vi "N4_201_Adjust.vi"(4 "Driver Name":T10, 5 "ValueIn":T7, 6 "Error Code":T11, 7 "Command":T7, 8 "error in":T9, 11 "DriverConnect in":T1={"InterfaceType"=enum."VISA", "OpenedSession"="", "InterfaceSettings"={"Interface"=enum."RS232", "EOS 4 read"=enum."LF (\\n)", "EOS 4 write"=enum."LF (\\n)", "TMO, ms"=10000, "Sett"=variant(cluster{"Baud Rate":u32, "Data Bits":u16, "Parity":u16, "Stop Bits":u16, "Flow Control":u16, "Eho":bool} {"Baud Rate"=75, "Data Bits"=0, "Parity"=0, "Stop Bits"=0, "Flow Control"=0, "Eho"=FALSE})}}) -> (0 "error out":T9, 3 "DriverConnect out":T1={"InterfaceType"=enum."VISA", "OpenedSession"="", "InterfaceSettings"={"Interface"=enum."RS232", "EOS 4 read"=enum."LF (\\n)", "EOS 4 write"=enum."LF (\\n)", "TMO, ms"=10000, "Sett"=variant(cluster{"Baud Rate":u32, "Data Bits":u16, "Parity":u16, "Stop Bits":u16, "Flow Control":u16, "Eho":bool} {"Baud Rate"=75, "Data Bits"=0, "Parity"=0, "Stop Bits"=0, "Flow Control"=0, "Eho"=FALSE})}})   [LabVIEW 2018]
uses:
  MOKO_LabViewLibrary/MokoLowLevel/MokoLowLovelControl/MLLC_ErrorCode.ctl
  MOKO_LabViewLibrary/MokoLowLevel/MokoLowLovelControl/MLLC_DriverName.ctl
  MOKO_LabViewLibrary/MokoLowLevel/MokoLowLovelControl/MLLC_Error.ctl
  MOKO_LabViewLibrary/MokoLowLevel/MokoLowLovelControl/MLLC_Boolean.ctl
  MOKO_LabViewLibrary/MokoLowLevel/MokoLowLovelControl/MLLC_Command.ctl
  MOKO_LabViewLibrary/MokoLowLevel/MokoLowLovelControl/MLLC_Delay.ctl
  MOKO_LabViewLibrary/MokoLowLevel/MokoLowLovelControl/MLLC_ConnectCluster.ctl
  MOKO_LabViewLibrary/MokoLowLevel/MokoLowLovelControl/MLLC_InterfaceType.ctl
  MOKO_LabViewLibrary/MokoLowLevel/MokoLowLovelControl/MLLC_OpenedSession.ctl
  MOKO_LabViewLibrary/MokoLowLevel/MokoLowLovelControl/MLLC_InterfaceSettings.ctl
  MOKO_LabViewLibrary/MokoLowLevel/MokoLowLovelControl/MLLC_InterfaceKind.ctl
panel:
  in  "step":T6
  in  "Sens":u32=1 caption="Точность\nнастройки" min=1 max=10 step=1 format="%.0dx"
  in  "Delay":dbl=500.0 caption="Задержка, \nмс" step=10.0
  out "timer":T6
  out "adjust event":T8
  in  "Value":dbl
  in  "OK Button":bool
  # "Откорректируйте значение Н4-101\n(c gпомощью скрола или кнопок вверх, вниз)"
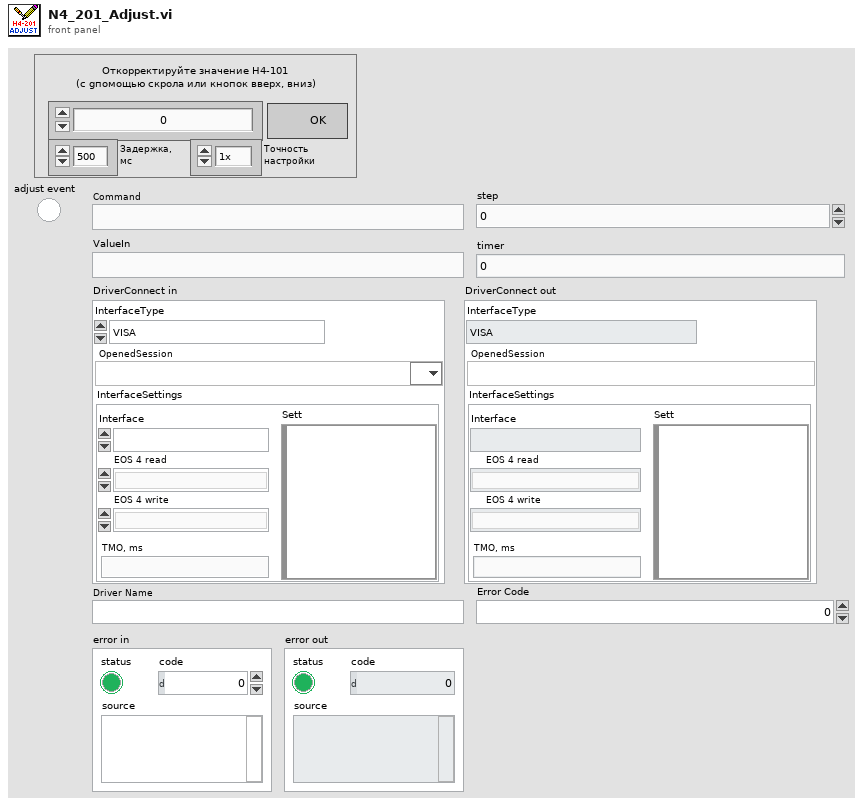
[diagram p1: front panel]
types:
  T1 = typedef "MLLC_ConnectCluster.ctl" = cluster{"InterfaceType":T2, "OpenedSession":T3, "InterfaceSettings":T4}
  T2 = typedef "MLLC_InterfaceType.ctl" = enum16{"VISA", "Prologix USB-GPIB"}
  T3 = typedef "MLLC_OpenedSession.ctl" = refnum<visa-resource-name>
  T4 = typedef "MLLC_InterfaceSettings.ctl" = cluster{"Interface":T5, "EOS 4 read":enum16{"Default (=EOS 4 write)", "CR (\\r)", "LF (\\n)", "None"}, "EOS 4 write":enum16{"CR+LF (\\r\\n)", "CR (\\r)", "LF (\\n)", "None"}, "TMO, ms":i32, "Sett":variant}
  T5 = typedef "MLLC_InterfaceKind.ctl" = enum16{"RS232", "GPIB", "USB", "Ethernet", "another"}
  T6 = typedef "MLLC_Delay.ctl" = dbl
  T7 = typedef "MLLC_Command.ctl" = string
  T8 = typedef "MLLC_Boolean.ctl" = bool
  T9 = typedef "MLLC_Error.ctl" = errorcluster
  T10 = typedef "MLLC_DriverName.ctl" = string
  T11 = typedef "MLLC_ErrorCode.ctl" = u32
  T12 = cluster{"button 1":bool, "button 2":bool, "button 3":bool, "button 4":bool}
  T13 = cluster{"Horizontal":i32, "Vertical":i32, "Scrolling":i32}
  T14 = cluster{"button 1":T8, "button 2":T8, "button 3":T8, "button 4":T8}
  T15 = typedef "eventvkey.ctl" = enum16{"ASCII", "Enter", "Return", "Shift", "Ctrl", "Alt", "Cmd", "Opt", "Caps", "NumLock", "Clear", "Break", "Up", "Down", "Left", "Right", "Insert", "Delete", "Home", "End", "PageUp", "PageDown", "Escape", "Help", "Pause", "ScrollLock", "F1", "F2", "F3", "F4", "F5", "F6", "F7", "F8", "F9", "F10", "F11", "F12", "F13", "F14", "F15", "F16", "F17", "F18", "F19", "F20", "F21", "F22", "F23", "F24", "Play", "VolumeUp", "VolumeDown", "Mute", "Two Byte Char"}
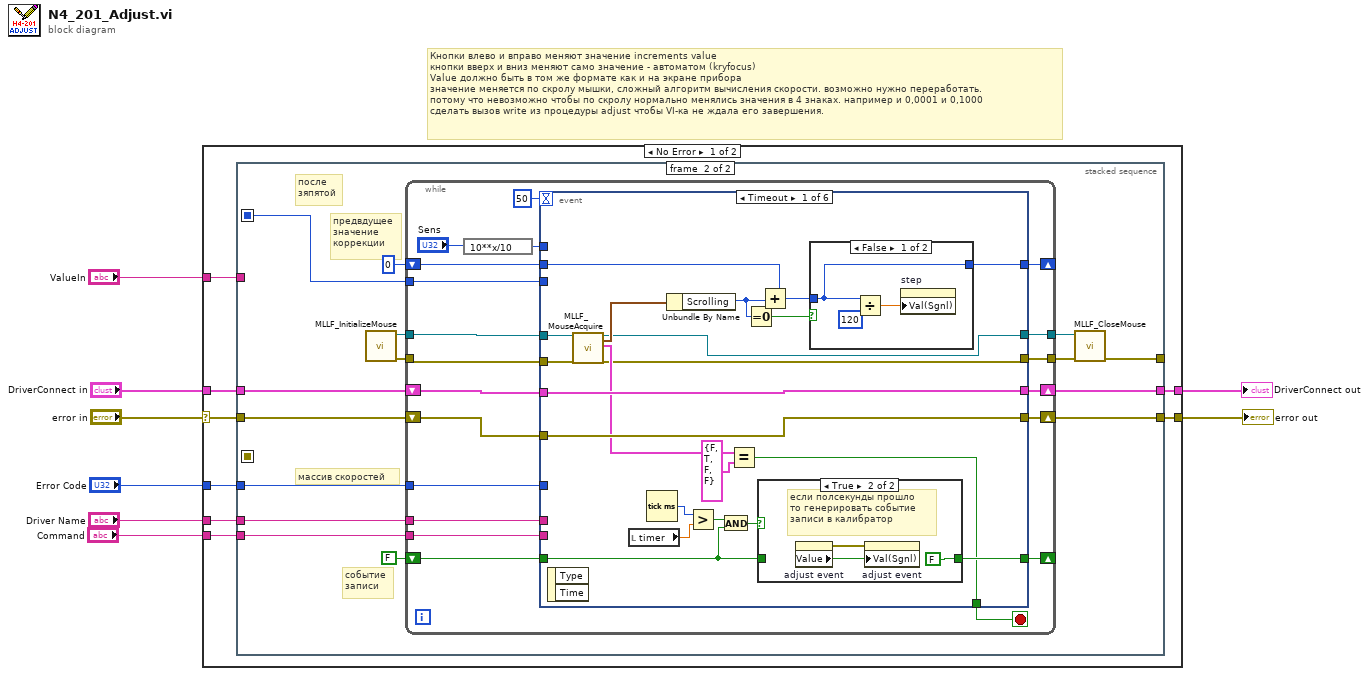
[diagram p0: block diagram]
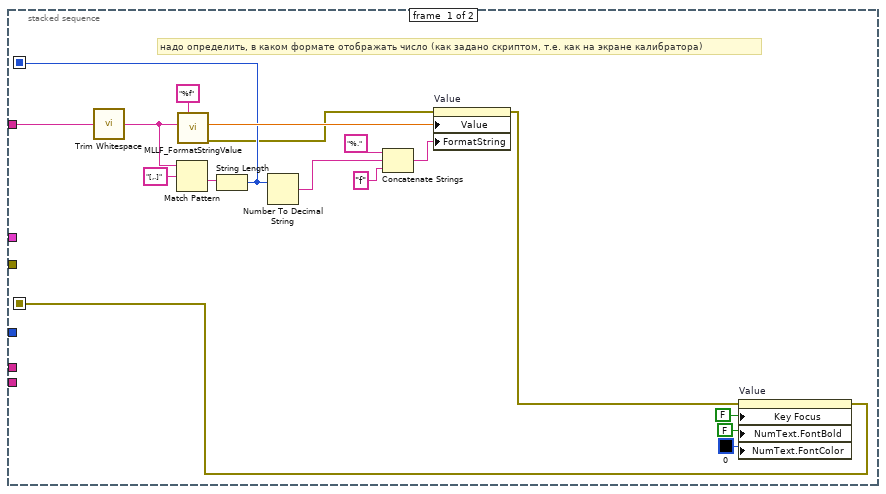
[diagram p2: hidden frame]
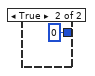
[diagram p3: hidden frame]
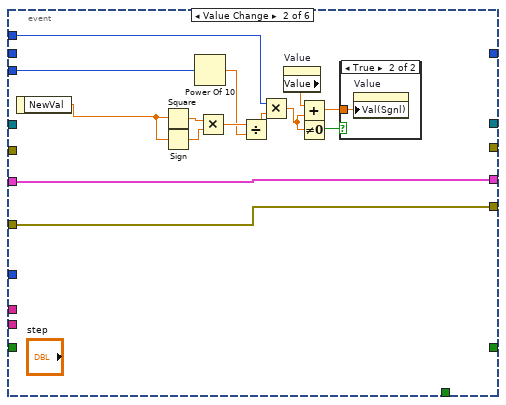
[diagram p5: hidden frame]
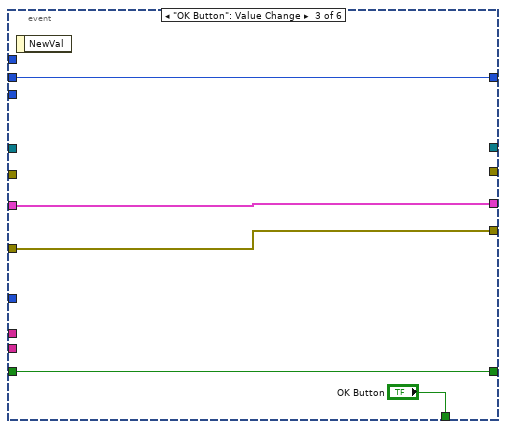
[diagram p7: hidden frame]
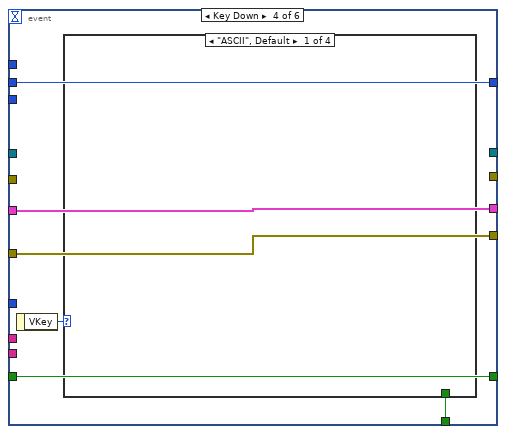
[diagram p8: hidden frame]
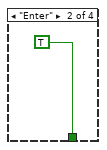
[diagram p9: hidden frame]
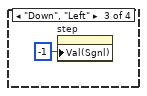
[diagram p10: hidden frame]
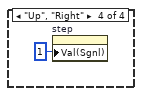
[diagram p11: hidden frame]
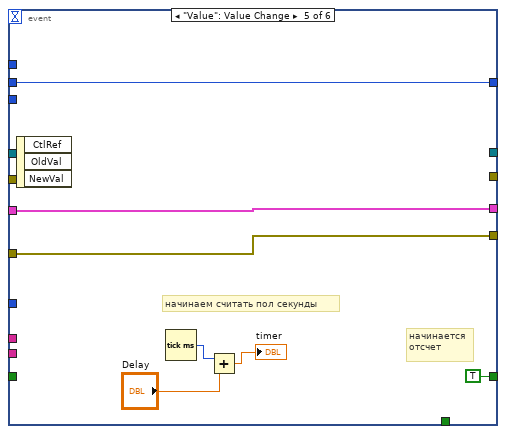
[diagram p12: hidden frame]
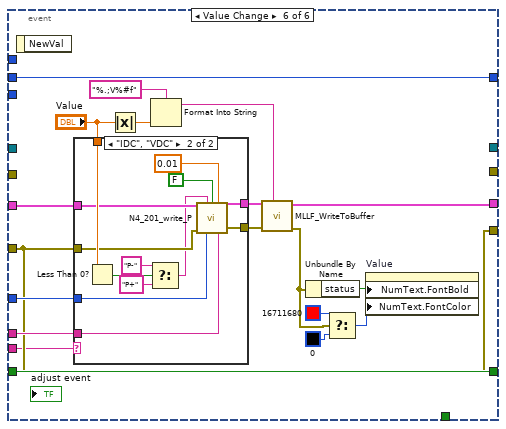
[diagram p13: hidden frame]
diagram:
  # "Кнопки влево и вправо меняют значение increments value\nкнопки вверх и вниз меняют само значение - автоматом (kryfocus)\nValue должно быть в том же формате как и на экране прибора\nзначение меняется по скролу мышки, сложный алгоритм вычисления скорости. возможно нужно переработать.\nпотому что невозможно чтобы по скролу нормально менялись значения в 4 знаках. например и 0,0001 и 0,1000\nсделать вызов write из процедуры adjust чтобы VI-ка не ждала его завершения."
  n1 = case shown="No Error" "error in" {
    selector: "error in" -> [w16 w169]
    tunnel: [w14 w169] -> w8
    tunnel: "Error Code" -> [w12 _]
    tunnel: "Driver Name" -> [w11 _]
    tunnel: "DriverConnect in" -> [w15 w168]
    tunnel: [w13 w168] -> w1
    tunnel: "ValueIn" -> [w10 _]
    tunnel: "Command" -> [w9 _]
    frame No Error {
      n2 = stacked-sequence {
        seq-local: [w23 _] -> [_ w41]
        seq-local: [w19 _] -> [_ _]
        tunnel: w16 -> [_ w34]
        tunnel: w15 -> [_ w35]
        tunnel: [_ w48] -> w14
        tunnel: [_ w47] -> w13
        tunnel: w12 -> [_ w37]
        tunnel: w11 -> [_ w36]
        tunnel: w10 -> [w18 _]
        tunnel: [_ w40] -> _
        tunnel: w9 -> [_ w38]
        frame #0 {
          # "надо определить, в каком формате отображать число (как задано скриптом, т.е. как на экране калибратора)"
          n3 = call <vilib>:"Trim Whitespace.vi"("string"=w18) -> ("trimmed string"=w17:string)  [unwired: 1 in]
          n4 = Match Pattern(string=w17, regular expression="[,.]") -> (after substring=w28:string)  [unwired: 1 in, 3 out]
          n5 = call "MLLF_FormatStringValue.vi"("String Value"=w17, "Format"="%f" ("format string")) -> ("error out"=w20:T9, "number"=w30:dbl)  [unwired: 7 in, 1 out]
          n6 = String Length(string=w28) -> (length=w23:i32)
          n7 = Number To Decimal String(number=w23) -> (decimal integer string=w24:string)  [unwired: 1 in]
          n8 = Concatenate Strings("%." ("format string"), w24, "f" ("format string")) -> (w25:string)
          n9 = property on="Value" class="DigNum (strict)"(error in=w20, "Value"=w30, "FormatString"=w25) -> (error out=w22:errorcluster)  [unwired: 1 in, 1 out]
          n10 = property on="Value" class="DigNum (strict)"(error in=w22, "Key Focus"=FALSE, "NumText.FontBold"=FALSE ("Numeric Text.Font:Bold"), "NumText.FontColor"=u32 0) -> (error out=w19:errorcluster)  [unwired: 1 in, 1 out]
        }
        frame #1 {
          # "массив скоростей"
          # "событие\nзаписи"
          # "предвдущее\nзначение\nкоррекции"
          # "после\nзяпятой"
          n11 = call "MLLF_InitializeMouse.vi"() -> ("error out"=w45:T9, "device ID"=w44:refnum<k1>)  [unwired: 10 in]
          n12 = while {
            shift-right: [w64] -> w48
            shift-left: w34 -> [w65]
            shift-right: [w63] -> w47
            shift-left: w35 -> [w66]
            tunnel: w37 -> [w62]
            tunnel: w36 -> [w61]
            shift-right: [w60] -> _
            shift-left: 0 -> [w59]
            tunnel: w45 -> [w49]
            tunnel: w44 -> [w50]
            tunnel: [w58] -> w43
            tunnel: [w57] -> w42
            tunnel: w41 -> [w56]
            shift-right: [w55] -> _
            shift-left: FALSE ("x > y?") -> [w54]
            tunnel: w38 -> [w53]
            stop <- w67 stop-if-true
            n13 = expression code="10**x/10"("Sens") -> (w52:u32)
            n14 = event shown="[0] Timeout" {
              selector: _ -> [_ _ _ _ _ _]
              dyn-events: _ -> [_ _ _ _ _ _]
              timeout: 50 -> [_ _ _ _ _ _]
              tunnel: [w77 _ "OK Button" w119 _ _] -> w67
              tunnel: w66 -> [w89 w111 w115 w121 w133 w146]
              tunnel: w65 -> [w88 w110 w116 w120 w132 w143]
              tunnel: [w88 w110 w116 w120 w132 w143] -> w64
              tunnel: [w89 w111 w115 w121 w133 w136] -> w63
              tunnel: w62 -> [_ _ _ _ _ w145]
              tunnel: w61 -> [_ _ _ _ _ w144]
              tunnel: [w79 _ w114 w123 w131 w149] -> w60
              tunnel: w59 -> [w81 _ w114 w123 w131 w149]
              tunnel: [w71 _ _ _ _ _] -> w58
              tunnel: [w72 _ _ _ _ _] -> w57
              tunnel: w56 -> [_ w99 _ _ _ _]
              tunnel: [w82 _ w113 w122 TRUE ("x > y?") w147] -> w55
              tunnel: w54 -> [w83 _ w113 w122 _ w147]
              tunnel: w53 -> [_ _ _ _ _ w140]
              tunnel: w52 -> [_ w100 _ _ _ _]
              tunnel: w50 -> [w73 _ _ _ _ _]
              tunnel: w49 -> [w70 _ _ _ _ _]
              event Timeout {
                n15 = event-data() -> ()  [unwired: 1 in, 2 out]
                n16 = call "MLLF_MouseAcquire.vi"("Device ID"=w73, "error in (no error)"=w70) -> ("Device ID"=w72:refnum<k1>, "Axis info"=w75:T13, "Button info"=w74:T14, "error out"=w71:T9)  [unwired: 14 in]
                n17 = local read "timer"() -> (w86:T6)
                n18 = Tick Count (ms)() -> (millisecond timer value=w87:u32)
                n19 = Unbundle By Name(w75) -> ("Scrolling"=w69:i32)
                n20 = Greater?(x=w87, y=w86) -> (0:w85:bool)
                n21 = And(x=w85, y=w83) -> (x .and. y?=w84:bool)
                n22 = Equal?(x=w74, y=T12 {"button 1"=FALSE, "button 2"=TRUE, "button 3"=FALSE, "button 4"=FALSE}) -> (x = y?=w77:bool)
                n23 = Equal To 0?(x=w69) -> (x = 0?=w76:bool)
                n24 = case shown="True" w84 {
                  tunnel: [w94 FALSE ("x > y?")] -> w82
                  tunnel: w83 -> [w94 _]
                  frame False {
                  }
                  frame True {
                    # "если полсекунды прошло\nто генерировать событие \nзаписи в калибратор"
                    n25 = property on="adjust event" class="Bool (strict)"() -> (error out=w96:errorcluster, "Value"=w97:bool)  [unwired: 2 in, 1 out]
                    n26 = property on="adjust event" class="Bool (strict)"(error in=w96, "Val(Sgnl)"=w97) -> ()  [unwired: 1 in, 2 out]
                  }
                }
                n27 = Add(x=w81, y=w69) -> (x+y=w80:i32)
                n28 = case shown="False" w76 {
                  tunnel: w80 -> [w90 _]
                  tunnel: [w90 0] -> w79
                  frame False {
                    n29 = Divide(x=w90, y=120) -> (x/y=w91:dbl)
                    n30 = property on="step" class="DigNum (strict)"("Val(Sgnl)"=w91) -> ()  [unwired: 2 in, 2 out]
                  }
                  frame True {
                  }
                }
              }
              event Value Change {
                n31 = event-data() -> ("NewVal"=w98:T6)  [unwired: 1 in]
                n32 = Square(x=w98) -> (x^2=w104:T6)
                n33 = Sign(1:w98) -> (0:w109:T6)
                n34 = Power Of 10(x=w99) -> (10^x=w103:dbl)
                n35 = Multiply(x=w104, y=w109) -> (x*y=w105:T6)
                n36 = Divide(x=w105, y=w103) -> (x/y=w102:T6)
                n37 = Multiply(x=w100, y=w102) -> (x*y=w101:T6)
                n38 = property on="Value" class="DigNum (strict)"() -> ("Value"=w108:dbl)  [unwired: 2 in, 2 out]
                n39 = Add(x=w108, y=w101) -> (x+y=w106:T6)
                n40 = Not Equal To 0?(x=w101) -> (x != 0?=w107:bool)
                n41 = case shown="True" w107 {
                  tunnel: w106 -> [_ w112]
                  frame False {
                  }
                  frame True {
                    n42 = property on="Value" class="DigNum (strict)"("Val(Sgnl)"=w112) -> ()  [unwired: 2 in, 2 out]
                  }
                }
              }
              event "OK Button": Value Change {
                n43 = event-data() -> ()  [unwired: 1 in, 1 out]
              }
              event Key Down {
                n44 = event-data() -> ("VKey"=w118:T15)  [unwired: 1 in]
                n45 = case shown="\"ASCII\", Default" w118 {
                  tunnel: [_ TRUE ("OK Button") _ _] -> w119
                  frame "ASCII", Default {
                  }
                  frame "Enter" {
                  }
                  frame "Down", "Left" {
                    n46 = property on="step" class="DigNum (strict)"("Val(Sgnl)"=i8 -1 ("Value (Signaling)")) -> ()  [unwired: 2 in, 2 out]
                  }
                  frame "Up", "Right" {
                    n47 = property on="step" class="DigNum (strict)"("Val(Sgnl)"=i8 1 ("Value (Signaling)")) -> ()  [unwired: 2 in, 2 out]
                  }
                }
              }
              event "Value": Value Change {
                # "начинается\nотсчет"
                # "начинаем считать пол секунды"
                n48 = event-data() -> ()  [unwired: 1 in, 3 out]
                n49 = Tick Count (ms)() -> (millisecond timer value=w130:u32)
                n50 = Add(x=w130, y="Delay") -> (x+y=→"timer":dbl)
              }
              event Value Change {
                n51 = event-data() -> ()  [unwired: 1 in, 1 out]
                n52 = case shown="\"IDC\", \"VDC\"" w140 {
                  tunnel: w146 -> [w154 w163]
                  tunnel: w145 -> [_ w161]
                  tunnel: w144 -> [_ w160]
                  tunnel: w143 -> [w153 w162]
                  tunnel: [w153 w157] -> w138
                  tunnel: [w154 w158] -> w139
                  tunnel: "Value" -> [_ w164]
                  frame "False", Default {
                  }
                  frame "IDC", "VDC" {
                    n53 = Less Than 0?(x=w164) -> (x < 0?=w165:bool)
                    n54 = Select(t="P-" ("String"), s=w165, f="P+" ("String")) -> (s? t:f=w159:string)
                    n55 = call "N4_201_write_P.vi"("DriverConnect in"=w163, "P"=w159, "RangeIsChanged?"=FALSE, "Command Time (s)"=0.01 ("Delay Time (s)"), "error in"=w162, "Error Code"=w161, "Driver Name"=w160) -> ("DriverConnect out"=w158:T1, "error out"=w157:T9)  [unwired: 7 in]
                  }
                }
                n56 = Absolute Value(x="Value") -> (abs(x)=w141:dbl)
                n57 = Format Into String(format string="%.;V%#f", w141) -> (resulting string=w137:string)  [unwired: 2 in, 1 out]
                n58 = call "MLLF_WriteToBuffer.vi"("String"=w137, "error in"=w138, "DriverConnect in"=w139) -> ("error out"=w134:T9, "DriverConnect out"=w136:T1)  [unwired: 5 in]
                n59 = Unbundle By Name(w134) -> ("status"=w135:bool)
                n60 = Select(t=u32 16711680, s=w134, f=u32 0) -> (s? t:f=w151:u32)
                n61 = property on="Value" class="DigNum (strict)"("NumText.FontBold"=w135, "NumText.FontColor"=w151) -> ()  [unwired: 2 in, 2 out]
              }
            }
          }
          n62 = call "MLLF_CloseMouse.vi"("error in (no error)"=w43, "device ID"=w42) -> ("error out"=w40:T9)  [unwired: 8 in]
        }
      }
    }
    frame Error {
    }
  }
  "error out" <- w8
  "DriverConnect out" <- w1
